vi "AODGlobals.vi"() -> ()   [LabVIEW 2017, in "AODControl.lvlib"]
uses:
  AODControl.lvlib
  AODControlFiles/InterfaceReferences.ctl
  AODControlFiles/LoadControl.ctl
  AODControlFiles/ExitButton.ctl
  MessageQueue/QueueOperations/All Message Queues.ctl
  MessageQueue/QueueOperations/Message Cluster.ctl
  MessageQueue/MessageQueue.lvlib
panel:
  in  "Are Ref. Initialized?":refnum<k4>
  out "Message Queues":T1
  in  "AOD Front Pannel References":T2
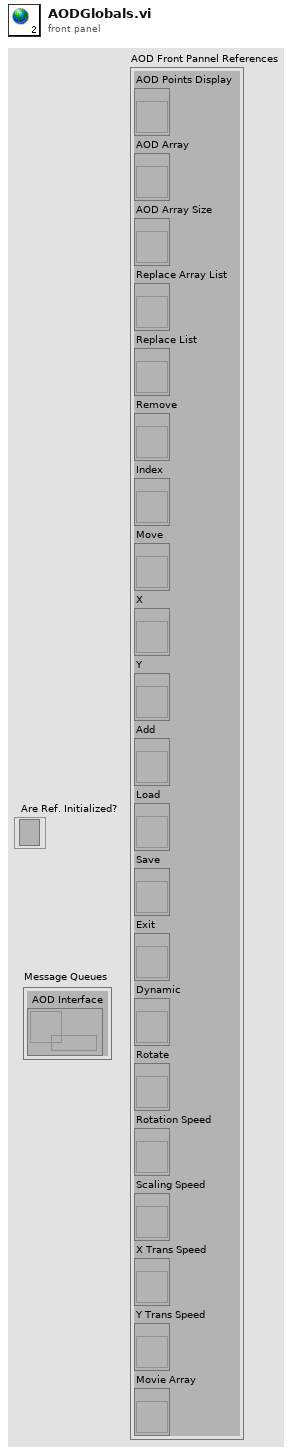
[diagram p1: front panel]
types:
  T1 = typedef "AODControl.lvlib/MessageQueue.lvlib/All Message Queues.ctl" = cluster{" AOD Interface":refnum<queue>}
  T2 = typedef "AODControl.lvlib/InterfaceReferences.ctl" = cluster{"AOD Points Display":refnum<vi>, "AOD Array":refnum<vi>, "AOD Array Size":refnum<vi>, "Replace Array List":refnum<vi>, "Replace List":refnum<vi>, "Remove":refnum<vi>, "Index":refnum<vi>, "Move":refnum<vi>, "X":refnum<vi>, "Y":refnum<vi>, "Add":refnum<vi>, "Load":refnum<vi>, "Save":refnum<vi>, "Exit":refnum<vi>, "Dynamic":refnum<vi>, "Rotate":refnum<vi>, "Rotation Speed":refnum<vi>, "Scaling Speed":refnum<vi>, "X Trans Speed":refnum<vi>, "Y Trans Speed":refnum<vi>, "Movie Array":refnum<vi>}
diagram:
